vi "Initialize.vi"(3 "Container State":T3, 4 "Previous State":variant, 5 "Previous Version":T2) -> (2 "Current State":T1={"Month"=1, "Day"=1, "Year"=2022})   [LabVIEW 2019, in "Custom Calendar.xctl"]
uses:
  Custom Calendar.xctl
  State.ctl
  <vilib>/_xctls/Container State.ctl
  <vilib>/_xctls/Version.ctl
  <vilib>/_xctls/XControlSupport.lvlib
panel:
  in  "Default Indicator State":T1={"Month"=1, "Day"=1, "Year"=2022}
  in  "Default Control State":T1={"Month"=1, "Day"=1, "Year"=2022}
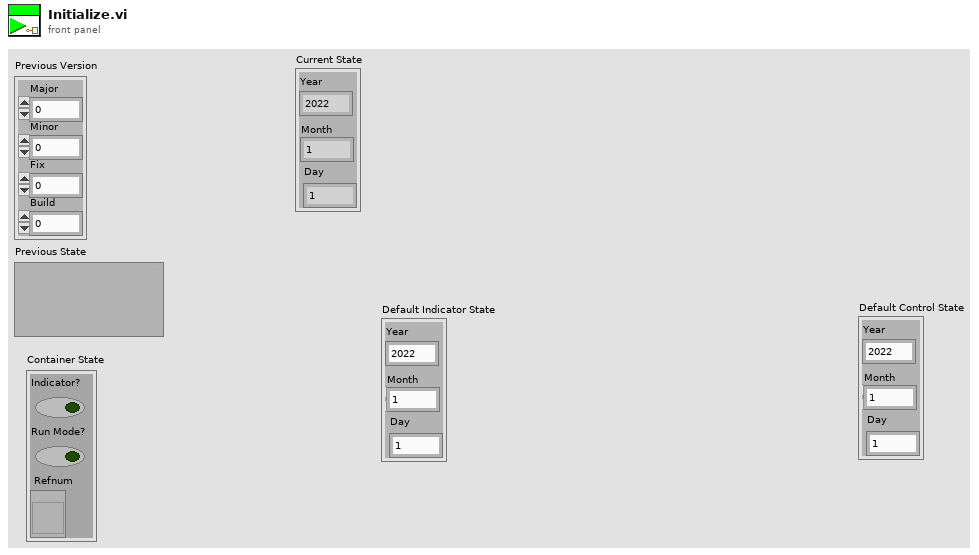
[diagram p1: front panel]
types:
  T1 = typedef "Custom Calendar.xctl/State.ctl" = cluster{"Month":i32, "Day":i32, "Year":i32}
  T2 = typedef "XControlSupport.lvlib/Version.ctl" = cluster{"Major":u16, "Minor":u16, "Fix":u16, "Build":u16}
  T3 = typedef "XControlSupport.lvlib/Container State.ctl" = cluster{"Indicator?":bool, "Run Mode?":bool, " Refnum":refnum<vi>}
  T4 = typedef "LVDateTimeRec.ctl" = cluster{"fractional second":dbl, "second":i32, "minute":i32, "hour":i32, "day of month":i32, "month":i32, "year":i32, "day of week":i32, "day of year":i32, "DST":i32}
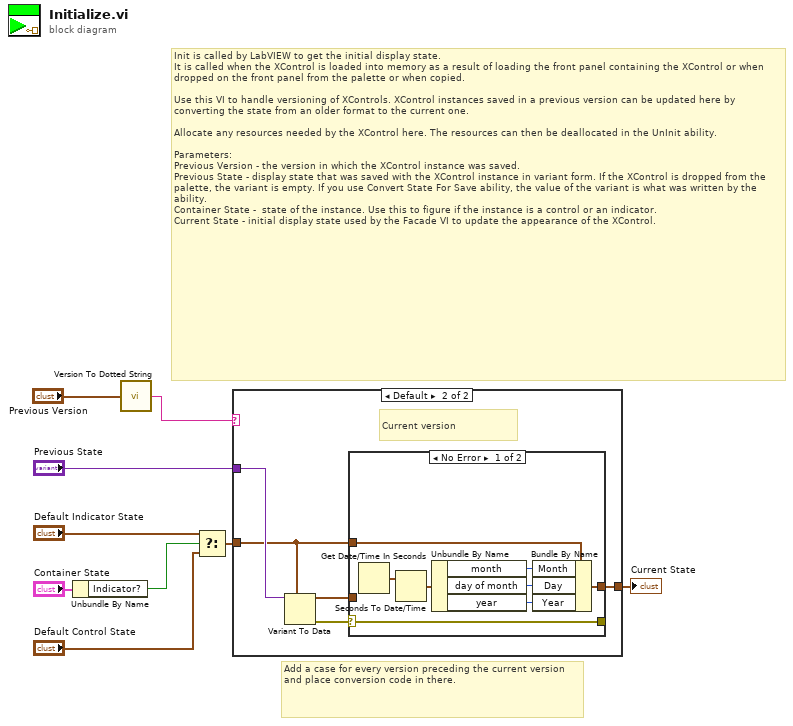
[diagram p0: block diagram]
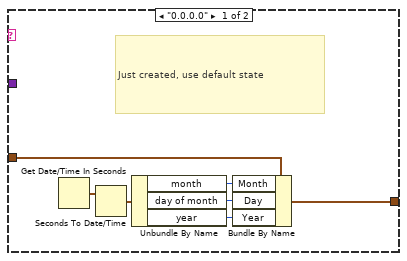
[diagram p2: hidden frame]
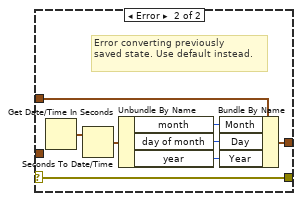
[diagram p3: hidden frame]
diagram:
  # "Add a case for every version preceding the current version and place conversion code in there."
  # "Init is called by LabVIEW to get the initial display state.\nIt is called when the XControl is loaded into memory as a result of loading the front panel containing the XControl or when dropped on the front panel from the palette or when copied.\n\nUse this VI to handle versioning of XControls. XControl instances saved in a previous version can be updated here by converting the state from an older format to the current one.\n\nAllocate any resources needed by the XControl here. The resources can then be deallocated in the UnInit ability.\n\nParameters:\nPrevious Version - the version in which the XControl instance was saved.\nPrevious State - display state that was saved with the XControl instance in variant form. If the XControl is dropped from the palette, the variant is empty. If you use Convert State For Save ability, the value of the variant is what was written by the ability. \nContainer State -  state of the instance. Use this to figure if the instance is a control or an indicator.\nCurrent State - initial display state used by the Facade VI to update the appearance of the XControl."
  n1 = Unbundle By Name("Container State") -> ("Indicator?"=w4:bool)
  n2 = call <vilib>:"Version To Dotted String.vi"("Version"="Previous Version") -> ("String Version"=w1:string)
  n3 = Select(t="Default Indicator State", s=w4, f="Default Control State") -> (s? t:f=w3:T1)
  n4 = case shown="Default" w1 {
    tunnel: "Previous State" -> [_ w21]
    tunnel: [w10 w17] -> w8
    tunnel: w3 -> [w11 w18]
    frame "0.0.0.0" {
      # "Just created, use default state"
      n5 = Get Date/Time In Seconds() -> (seconds since 1Jan1904=w16:timestamp)
      n6 = Seconds To Date/Time(time stamp (now)=w16) -> (date time rec=w15:T4)  [unwired: 1 in]
      n7 = Unbundle By Name(w15) -> ("month"=w14:i32, "day of month"=w13:i32, "year"=w12:i32)
      n8 = Bundle By Name(cluster=w11, "Month"=w14, "Day"=w13, "Year"=w12) -> (w10:T1)
    }
    frame Default {
      # "Current version"
      n9 = Variant To Data(type=w18, Variant=w21) -> (data=w19:T1, error out=w20:errorcluster)  [unwired: 1 in]
      n10 = case shown="No Error" w20 {
        selector: w20 -> [w29 w37]
        tunnel: w19 -> [_ _]
        tunnel: [w22 w31] -> w17
        tunnel: w18 -> [w23 w32]
        tunnel: [w29 w37] -> _
        frame No Error {
          n11 = Get Date/Time In Seconds() -> (seconds since 1Jan1904=w28:timestamp)
          n12 = Seconds To Date/Time(time stamp (now)=w28) -> (date time rec=w27:T4)  [unwired: 1 in]
          n13 = Unbundle By Name(w27) -> ("month"=w26:i32, "day of month"=w25:i32, "year"=w24:i32)
          n14 = Bundle By Name(cluster=w23, "Month"=w26, "Day"=w25, "Year"=w24) -> (w22:T1)
        }
        frame Error {
          # "Error converting previously \nsaved state. Use default instead."
          n15 = Get Date/Time In Seconds() -> (seconds since 1Jan1904=w36:timestamp)
          n16 = Seconds To Date/Time(time stamp (now)=w36) -> (date time rec=w35:T4)  [unwired: 1 in]
          n17 = Unbundle By Name(w35) -> ("month"=w30:i32, "day of month"=w34:i32, "year"=w33:i32)
          n18 = Bundle By Name(cluster=w32, "Month"=w30, "Day"=w34, "Year"=w33) -> (w31:T1)
        }
      }
    }
  }
  "Current State" <- w8
